vi "Set Process Kill timeout.vi"(8 "error in (no error)":errorcluster, 10 "Process Kill timeout (500 ms)":i32=500 caption="timeout", 11 "SMO in":refnum<class "SMO.lvclass">) -> (0 "error out":errorcluster, 3 "SMO out":refnum<class "SMO.lvclass">)   [LabVIEW 2013, in "SMO.lvclass"]
uses:
  SMO.lvclass
  SMO.lvclass/SMO.ctl
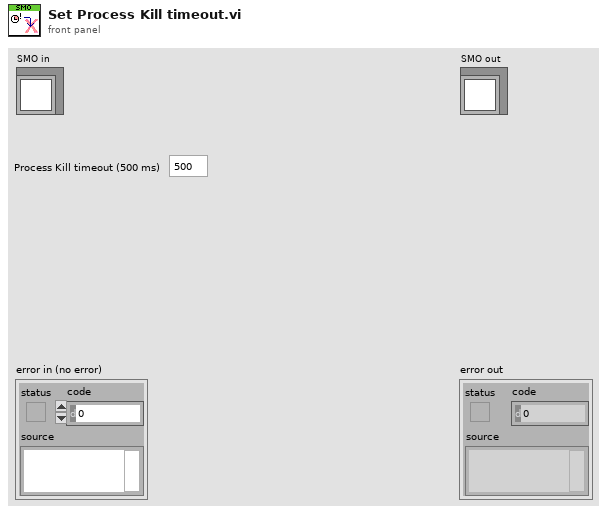
[diagram p1: front panel]
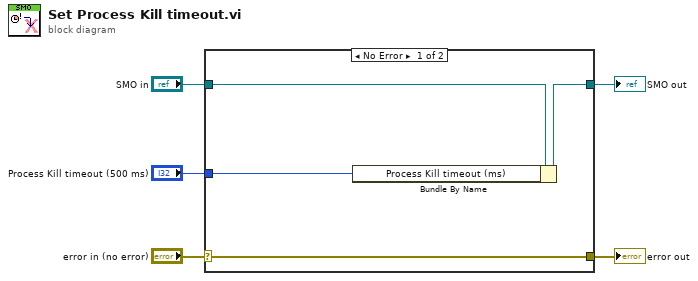
[diagram p0: block diagram]
diagram:
  n1 = case shown="No Error" "error in (no error)" {
    selector: "error in (no error)" -> [w9 w10]
    tunnel: [w9 w10] -> w4
    tunnel: [w6 w11] -> w2
    tunnel: "SMO in" -> [w8 w11]
    tunnel: "Process Kill timeout (500 ms)" -> [w7 _]
    frame No Error {
      n2 = Bundle By Name(cluster=w8, "Process Kill timeout (ms)"=w7) -> (w6:refnum<class "SMO.lvclass">)
    }
    frame Error {
    }
  }
  "error out" <- w4
  "SMO out" <- w2
